vi "HFRR ADV v025 new software.vi"() -> ()   [LabVIEW 2025] (continued)
                    n3885 = local read item#-1() -> (w5335)
                    n3886 = Number To Fractional String(number=w5335, width (-)=i16 10, precision (6)=i16 4) -> (F-format string=w5339:string)  [unwired: 1 in]
                    n3887 = Concatenate Strings("LinearDeformation\":\"", w5339, w5337) -> (w5336:string)
                  }
                  frame #5 {
                    n3888 = local read "AIR TEMP"() -> (w5342:dbl)
                    n3889 = local read "Json St Flg"() -> (w5344:bool)
                    n3890 = local read "Json End Flg"() -> (w5345:bool)
                    n3891 = Number To Fractional String(number=w5342, width (-)=i16 10, precision (6)=i16 4) -> (F-format string=w5348:string)  [unwired: 1 in]
                    n3892 = Concatenate Strings("Vibration\":\"", w5348, w5346) -> (w5343:string)
                    n3893 = And(x=w5344, y=w5345) -> ()  [unwired: 1 out]
                  }
                  frame #6 {
                    n3894 = local read "Json End Flg"() -> (w5352:bool)
                    n3895 = Get Date/Time In Seconds() -> (seconds since 1Jan1904=w5360:timestamp)
                    n3896 = local read "Json St Flg"() -> (w5351:bool)
                    n3897 = To Double Precision Float(number=w5360) -> (double precision float=w5359:dbl)
                    n3898 = Subtract(x=w5359, y=2082844800.0) -> (x-y=w5357:dbl)
                    n3899 = Number To Fractional String(number=w5357, width (-)=i16 12, precision (6)=i16 0) -> (F-format string=w5354:string)  [unwired: 1 in]
                    n3900 = case shown="True" w5352 {
                      tunnel: ["" w5367] -> w5361
                      tunnel: w5354 -> [_ w5368]
                      tunnel: w5353 -> [_ w5366]
                      frame False {
                      }
                      frame True {
                        n3901 = local write "Json End Flg"(FALSE ("Json St Flg")) -> ()
                        n3902 = Concatenate Strings("End\": \"", w5368, w5366) -> (w5367:string)
                      }
                    }
                    n3903 = case shown="True" w5351 {
                      tunnel: [w5371 w5374] -> w5362
                      tunnel: w5354 -> [_ w5375]
                      tunnel: w5353 -> [_ w5372]
                      frame False {
                        n3904 = local read "St Str"() -> (w5371:string)
                      }
                      frame True {
                        n3905 = Concatenate Strings("Start\":\"", w5375, w5372) -> (w5374:string)
                        "St Str" <- w5374
                        n3906 = local write "Json St Flg"(FALSE ("Json St Flg")) -> ()
                      }
                    }
                    n3907 = Concatenate Strings(w5362, w5361, w5364) -> (w5363:string)
                  }
                }
                n3908 = local read "FILE"() -> (w5232:string)
                n3909 = Concatenate Strings("\",\"OperatorID\":\"" ("string"), "Operator ID") -> (w5235:string)
                n3910 = Concatenate Strings("\",\"DatasetTitle\":\"" ("string"), w5232) -> (w5234:string)
                n3911 = Concatenate Strings("\",\"SerialNumber\":\"" ("string"), "Serial No") -> (w5264:string)
                n3912 = Concatenate Strings("\",\"ModelNumber\":\"" ("string"), "Model No") -> (w5263:string)
                n3913 = Concatenate Strings(w5264, w5263) -> (w5246:string)
                n3914 = Concatenate Strings("{\"SecretKey\":\"", "Secret Key", w5246, w5235, w5234, "\",\"Samples\":[") -> (w5251:string)
                n3915 = Concatenate Strings(w5253, w5257, w5256, w5255, w5254, w5238, w5239, w5240) -> (w5252:string)
                n3916 = Concatenate Strings(w5251, w5252, "]}") -> (w5250:string)
                n3917 = stacked-sequence {
                  tunnel: w5250 -> [w5279 _ _]
                  tunnel: [_ _ w5296] -> _
                  frame #0 {
                    (unwired) FALSE ("convert eol (F)")
                    w5281 = enum16{"start", "end", "current"}."start" ("pos mode (0:2)")
                    n3918 = Path To String(path="Path") -> (string=w5287:string)
                    n3919 = Concatenate Strings(w5287, "\\", "Data File Name") -> (w5289:string)
                    n3920 = local write "standard output"(" ") -> ()
                    n3921 = String To Path(string=w5289) -> (path=w5278:path)
                    n3922 = call <vilib>:"Open_Create_Replace File.vi"("advisory dialog? (display:T)"=FALSE, "function (open:0)"=T30."create or replace", "file path"=w5278) -> ("error out"=w5292:errorcluster, "refnum"=w5291:refnum<file>)  [unwired: 5 in, 2 out]
                    n3923 = Set File Position(refnum=w5291, from (0:start)=w5281, error in=w5292) -> (refnum out=w5272:refnum<file>, error out=w5271:errorcluster)  [unwired: 1 in]
                    n3924 = Write to Binary File(file (use dialog)=w5272, data=" ", error in=w5271, 5:FALSE ("prepend array or string size? (T)")) -> (refnum out=w5282:refnum<file>, error out=w5283:errorcluster)  [unwired: 2 in, 1 out]
                    n3925 = Set File Position(offset (in bytes) (0)=w5281, refnum=w5282, error in=w5283) -> (refnum out=w5275:refnum<file>, error out=w5274:errorcluster)  [unwired: 1 in]
                    n3926 = Write to Binary File(file (use dialog)=w5275, data=w5279, error in=w5274, 5:FALSE ("prepend array or string size? (T)")) -> (error out=w5277:errorcluster)  [unwired: 2 in, 2 out]
                    n3927 = flat-sequence {
                      tunnel: w5278 -> [w5294]
                      tunnel: w5277 -> [_]
                      frame #0 {
                        n3928 = call <vilib>:"Read Characters From File.vi"("file path (dialog if empty)"=w5294) -> ("character string"=→"JSON string":string)  [unwired: 5 in, 3 out]
                      }
                    }
                    "SinglePoint" <- w5279
                  }
                  frame #1 {
                  }
                  frame #2 {
                    (unwired) "\"Stored\": true" ("string")
                    n3929 = call <vilib>:"System Exec.vi"("run minimized? (F)"=TRUE, "wait until completion? (T)"=TRUE, "working directory"=path "C:/LAB-IQ-NXT", "command line"="C:\\LAB-IQ-NXT\\JPost.bat") -> ("standard error"=→"Respose From Server":string, "standard output"=w5299:string)  [unwired: 4 in, 2 out]
                    "standard output" <- w5299
                    n3930 = Match Pattern(string=w5299, regular expression="JSON Check String") -> (match substring=w5297:string, offset past match=w5296:i32)  [unwired: 1 in, 2 out]
                    n3931 = Equal?(x=w5297, y="JSON Check String") -> (x = y?=→"Upload \nConfirmed":bool)
                  }
                }
              }
            }
            n3932 = local read "Quit"() -> (w5220:bool)
          }
        }
      }
    }
    frame Enabled {
    }
  }
  n3933 = disable-structure shown="Disabled" {
    disable-tunnel: _ -> [w5382 _]
    frame Disabled {
      n3934 = while {
        shift-right: [w5390] -> w5378
        shift-left: _ -> [w5391]
        shift-right: [w5388] -> w5379
        shift-left: errorcluster {"status"=TRUE, "code"=0, "source"="Init"} ("error out") -> [w5389]
        shift-right: [w5386] -> _
        shift-left: "" -> [w5387]
        tunnel: [w5384] -> _
        tunnel: w5382 -> [_]
        i -> [w5384]
        stop <- w5383 stop-if-true
        n3935 = flat-sequence {
          tunnel: [w5392] -> w5385
          frame #0 {
            n3936 = Wait (ms)(milliseconds to wait=10.0 ("Delay")) -> (millisecond timer value=w5392:u32)
          }
        }
        n3937 = case shown="No Error" w5389 {
          selector: w5389 -> [w5422 w5541]
          tunnel: [w5405 w5543] -> w5390
          tunnel: [w5404 w5542] -> w5388
          tunnel: w5391 -> [w5423 w5535]
          tunnel: w5387 -> [w5403 w5534]
          tunnel: [w5402 w5534] -> w5386
          tunnel: w5385 -> [_ _]
          frame No Error {
            n3938 = Concatenate Strings("\r", "\n") -> (w5414:string)  [unwired: 1 in]
            n3939 = case shown="True" w5415 {
              tunnel: w5423 -> [w5447 w5454]
              tunnel: w5422 -> [w5446 w5453]
              tunnel: [w5447 w5452] -> w5421
              tunnel: [w5446 w5451] -> w5401
              tunnel: w5414 -> [_ w5450]
              frame False {
              }
              frame True {
                n3940 = VISA Write(VISA resource name=w5454, write buffer=w5450, error in (no error)=w5453) -> (VISA resource name out=w5452:refnum<visa-resource-name>, error out=w5451:errorcluster)  [unwired: 1 out]
                n3941 = local write "Read String"("") -> ()
                n3942 = local write item#-1(FALSE) -> ()
              }
            }
            n3943 = property class="Instr"(reference=w5421, error in=w5401) -> (reference out=w5420:refnum<visa-resource-name>, error out=w5419:errorcluster, "Serial Settings:Number of Bytes at Serial Port"=w5418:u32)
            n3944 = Greater?(x=w5418, y=u32 100) -> (0:w5416:bool)
            n3945 = case shown="True" w5416 {
              tunnel: w5420 -> [w5457 w5481]
              tunnel: w5419 -> [w5456 w5480]
              tunnel: w5418 -> [_ w5479]
              tunnel: [w5457 w5478] -> w5407
              tunnel: [w5456 w5477] -> w5406
              tunnel: w5403 -> [w5455 w5476]
              tunnel: [w5455 ""] -> w5402
              frame False {
              }
              frame True {
                w5466 = u32 6 ("y")
                # "Page 84 of \nmanual"
                n3946 = VISA Read(VISA resource name=w5481, byte count=w5479, error in (no error)=w5480) -> (VISA resource name out=w5478:refnum<visa-resource-name>, read buffer=w5474:string, error out=w5477:errorcluster)  [unwired: 1 out]
                n3947 = while {
                  tunnel: w5474 -> [w5530]
                  tunnel: [w5526] -> w5468 mode=indexing
                  tunnel: [w5520] -> w5472 mode=indexing
                  tunnel: [w5518] -> _
                  i -> [w5518]
                  stop <- w5523 stop-if-true
                  n3948 = String Subset(string=w5530, offset (0)=w5518) -> (substring=w5525:string)  [unwired: 1 in]
                  n3949 = String To Byte Array(string=w5525) -> (unsigned byte array=w5529:u8[])
                  n3950 = String Length(string=w5525) -> (length=w5524:i32)
                  n3951 = Index Array(array=w5529) -> (element=w5528:u8)  [unwired: 1 in]
                  n3952 = Equal To 0?(x=w5524) -> (x = 0?=w5523:bool)
                  n3953 = Number To Boolean Array(number=w5528) -> (Boolean array=w5522:bool[])
                  n3954 = Reverse 1D Array(array=w5522) -> (reversed array=w5521:bool[])
                  n3955 = And(x=w5522, y=bool[] [FALSE, FALSE, FALSE, FALSE, FALSE, FALSE, TRUE, TRUE] ("Boolean array")) -> (x .and. y?=w5526:bool[])
                  n3956 = And(x=w5521, y=bool[] [FALSE, FALSE, TRUE, TRUE, TRUE, TRUE, TRUE, TRUE] ("Boolean array")) -> (x .and. y?=w5520:bool[])
                }
                n3957 = Concatenate Strings(w5476, w5474) -> (→"Read String":string)
                n3958 = while {
                  tunnel: w5468 -> [w5517] mode=indexing
                  tunnel: [w5513] -> w5471
                  i -> [w5513]
                  stop <- w5514 stop-if-true
                  n3959 = Search 1D Array(1D array=w5517, element=TRUE) -> (index of element=w5515:i32)  [unwired: 1 in]
                  n3960 = Less Than 0?(x=w5515) -> (x < 0?=w5514:bool)
                }
                n3961 = Delete From Array(array=w5472, length=w5471, index (row)=0) -> (array with subset deleted=w5467:bool[][])  [unwired: 1 in, 1 out]
                n3962 = Array Size(array=w5467) -> (size(s)=w5469:i32[])
                n3963 = Index Array(array=w5469) -> (element=w5461:i32)  [unwired: 1 in]
                n3964 = Greater?(x=w5461, y=w5466) -> (0:w5464:bool)
                n3965 = Subtract(x=w5461, y=w5466) -> (x-y=w5465:u32)
                n3966 = Select(t=w5465, s=w5464, f=u32 0) -> (s? t:f=w5462:u32)
                n3967 = while {
                  tunnel: w5467 -> [w5500]
                  tunnel: [w5502] -> w5460 mode=indexing
                  tunnel: w5462 -> [w5484]
                  i -> [w5501]
                  stop <- w5499 stop-if-true
                  w5491 = 6 ("index")
                  w5490 = 2 ("length")
                  # "Page 65 of \nmanual"
                  n3968 = Multiply(x=u32 3 ("y"), y=w5501) -> (x*y=w5498:u32)
                  n3969 = Divide(x=u32 102 ("y"), y=u32 65520) -> (x/y=w5508:dbl)
                  n3970 = Greater Or Equal?(x=w5498, y=w5484) -> (x >= y?=w5499:bool)
                  n3971 = Index Array(array=w5500, index (row) #1=w5498) -> (element #1=w5496:bool[], element #2=w5495:bool[], element #3=w5494:bool[])  [unwired: 5 in]
                  n3972 = Reverse 1D Array(array=w5496) -> (reversed array=w5489:bool[])
                  n3973 = Reverse 1D Array(array=w5495) -> (reversed array=w5493:bool[])
                  n3974 = Reverse 1D Array(array=w5494) -> (reversed array=w5492:bool[])
                  n3975 = Delete From Array(array=w5489, length=w5490, index=w5491) -> (array with subset deleted=w5485:bool[])  [unwired: 1 out]
                  n3976 = Delete From Array(array=w5493, length=w5490, index=w5491) -> (array with subset deleted=w5486:bool[])  [unwired: 1 out]
                  n3977 = Delete From Array(array=w5492, length=w5490, index=w5491) -> (array with subset deleted=w5487:bool[])  [unwired: 1 out]
                  n3978 = Insert Into Array(array=bool[] [] ("Boolean array"), new element #1=w5485, new element #2=w5486, new element #3=w5487) -> (w5488:bool[])  [unwired: 1 in]
                  n3979 = Boolean Array To Number(Boolean array=w5488) -> (number=w5497:u32)
                  n3980 = Multiply(x=w5508, y=w5497) -> (x*y=w5507:dbl)
                  n3981 = Decrement(x=w5507) -> (x-1=w5506:dbl)
                  n3982 = Divide(x=w5506, y=u32 100) -> (x/y=w5504:dbl)
                  n3983 = Multiply(x=w5504, y=u32 10) -> (x*y=w5502:dbl)
                }
                n3984 = Delete From Array(array=w5460) -> (array with subset deleted=w5459:dbl[])  [unwired: 2 in, 1 out]
                "Waveform Graph 5" <- w5459
                "Waveform Chart 3" <- w5459
                n3985 = call-poly <vilib>:"Mean.vi"("X"=w5459) -> ("mean"=w5458:dbl)  [unwired: 1 out]
                n3986 = case shown="True" {
                  selector: _ -> [_ _]
                  tunnel: w5458 -> [_ w5483]
                  frame False {
                  }
                  frame True {
                    n3987 = local write item#-1(FALSE ("Zero 4")) -> ()
                    "z_measure" <- w5483
                  }
                }
              }
            }
            n3988 = local read item#-1() -> (w5398)
            n3989 = local read item#-1() -> (w5397)
            n3990 = local read item#-1() -> (w5399)
            n3991 = local read item#-1() -> (w5396)
            n3992 = case shown="True" w5394 {
              tunnel: w5398 -> [_ w5426]
              tunnel: w5399 -> [_ w5425]
              frame False {
              }
              frame True {
                n3993 = Build Array(w5426, w5425) -> (w5424:void[])
                n3994 = local read item#-1() -> (w5429)
                n3995 = Build Array (concatenate)(w5429, w5424) -> (w5427:void[])
                n3996 = local write item#-1(w5427) -> ()
                n3997 = local write item#-1(FALSE ("Boolean 8")) -> ()
              }
            }
            n3998 = call "Build XY Graph"("Enable"=w5396, "Reset"=w5397, "Y Input"=w5399, "X Input"=w5398) -> ("XY Graph"=w5395:cluster{"Y":dbl[], "Y":dbl[]}[])  [unwired: 6 in, 1 out]
            n3999 = case shown="True" {
              selector: _ -> [_ _]
              frame False {
              }
              frame True {
                n4000 = local read item#-1() -> (w5430)
                n4001 = Index Array(array=w5430, index (col) #1=0 ("disabled index (col)"), index (col) #2=1 ("index (col)")) -> (element #1=w5432, element #2=w5431)  [unwired: 2 in]
                n4002 = call <vilib>:"Linear Fit.vi"("Y"=w5432, "X"=w5431) -> ()  [unwired: 9 in, 5 out]
                n4003 = local write item#-1(FALSE ("Boolean 9")) -> ()
              }
            }
            n4004 = case shown="True" {
              selector: _ -> [_ _]
              frame False {
              }
              frame True {
                n4005 = local write item#-1(dbl[][] [] ("Captured Values")) -> ()
                n4006 = local write item#-1(FALSE ("Boolean 7")) -> ()
              }
            }
            n4007 = Concatenate Strings("\r", "\n") -> (w5409:string, w5408:string)
            n4008 = case shown="True" w5400 {
              tunnel: w5407 -> [w5439 w5445]
              tunnel: w5406 -> [w5438 w5444]
              tunnel: [w5439 w5443] -> w5405
              tunnel: [w5438 w5442] -> w5404
              tunnel: w5409 -> [_ w5441]
              frame False {
              }
              frame True {
                n4009 = VISA Write(VISA resource name=w5445, write buffer=w5441, error in (no error)=w5444) -> (VISA resource name out=w5443:refnum<visa-resource-name>, error out=w5442:errorcluster)  [unwired: 1 out]
                n4010 = local write item#-1(FALSE ("WRITE")) -> ()
              }
            }
          }
          frame Error {
            w5533 = u16 10 items=["1.0"=10, "1.5"=15, "2.0"=20] ("stop bits (10: 1 bit)")
            n4011 = Wait (ms)(milliseconds to wait=u32 20) -> ()  [unwired: 1 out]
            n4012 = VISA Close(VISA resource name=w5535, error in (no error)=w5541) -> (error out=w5540:errorcluster)
            n4013 = call <vilib>:"Clear Errors.vi"("error in (no error)"=w5540) -> ("error out"=w5539:errorcluster)  [unwired: 5 in, 1 out]
            n4014 = call-poly "VISA Configure Serial Port"("timeout (10sec)"=u32 200, "Enable Termination\nChar (T)"=TRUE ("Enable Termination\nChar (T)"), "baud rate (9600)"=u32 921600, "error in (no error)"=w5539, "stop bits (10: 1 bit)"=w5533) -> ("VISA resource name"=w5531:refnum<visa-resource-name>, "VISA resource name out"=w5543:refnum<visa-resource-name>, "error out"=w5542:errorcluster)  [unwired: 8 in]
          }
        }
        n4015 = local read "Quit"() -> (w5383:bool)
      }
      n4016 = VISA Close(VISA resource name=w5378, error in (no error)=w5379) -> (error out=w5377:errorcluster)
      n4017 = call <vilib>:"Clear Errors.vi"("error in (no error)"=w5377) -> ()  [unwired: 5 in, 2 out]
    }
    frame Enabled {
    }
  }
  n4018 = disable-structure shown="Disabled" {
    disable-tunnel: _ -> [w5548 _]
    frame Disabled {
      n4019 = while {
        tunnel: [w5555] -> _
        shift-right: [w5552] -> w5545
        shift-left: _ -> [w5554]
        shift-right: [w5553] -> w5546
        shift-left: errorcluster {"status"=TRUE, "code"=0, "source"="Init"} ("error out") -> [w5551]
        tunnel: w5548 -> [_]
        i -> [w5555]
        stop <- w5549 stop-if-true
        n4020 = flat-sequence {
          tunnel: w5551 -> [w5646]
          tunnel: [w5646] -> w5550
          frame #0 {
            n4021 = Wait (ms)(milliseconds to wait=u32 50) -> ()  [unwired: 1 out]
          }
        }
        n4022 = case shown="No Error" w5550 {
          selector: w5550 -> [w5596 w5639]
          tunnel: w5554 -> [w5595 w5638]
          tunnel: [w5562 w5629] -> w5553
          tunnel: [w5563 w5637] -> w5552
          frame No Error {
            w5589 = T31 {"Mode"=enum."RTU", "Slave Address"=1} ("Serial Parameters")
            n4023 = call-poly <vilib>:"MB Serial Master Query (poly).vi"("VISA resource name"=w5595, "Starting Address"=i16 1000, "Quantity"=u16 1, "Timeout"=u32 1000, "error in"=w5596, "Serial Parameters"=w5589) -> ("VISA resource name out"=w5590:refnum<visa-resource-name>, "Input Registers"=w5592:u16[], "error out"=w5588:errorcluster)  [unwired: 10 in, 1 out]
            n4024 = Random Number (0-1)() -> (number: 0 to 1=w5577:dbl)
            n4025 = Index Array(array=w5592, index=0) -> (element=w5587:u16)
            n4026 = Subtract(x=w5577, y=0.5) -> (x-y=w5576:dbl)
            n4027 = Divide(x=w5587, y=10 ("index")) -> (x/y=w5581:dbl)
            n4028 = Multiply(x=w5576, y=0.5) -> (x*y=w5575:dbl)
            n4029 = Add(x=w5581, y=w5575) -> (x+y=w5580:dbl)
            n4030 = local read "Amb temp"() -> (w5564:dbl)
            n4031 = Multiply(x=w5580, y=0.2) -> (x*y=w5584:dbl)
            n4032 = Multiply(x=w5564, y=0.8) -> (x*y=w5582:dbl)
            n4033 = Add(x=w5584, y=w5582) -> (x+y=w5565:dbl)
            n4034 = local read "set temp old"() -> (w5559:dbl)
            n4035 = local write "Amb temp"(w5565) -> ()
            n4036 = Select(t="SetTemp 2", s="Heater", f=100.0) -> (s? t:f=w5560:dbl)
            n4037 = Not Equal?(x=w5560, y=w5559) -> (x != y?=w5558:bool)
            n4038 = case shown="True" w5558 {
              tunnel: w5590 -> [w5624 w5626]
              tunnel: [w5623 w5626] -> w5570
              tunnel: w5588 -> [w5622 w5625]
              tunnel: [w5621 w5625] -> w5568
              tunnel: w5560 -> [w5616 _]
              tunnel: w5589 -> [w5618 w5627]
              tunnel: [w5618 w5627] -> w5571
              frame True {
                n4039 = Multiply(x=w5616, y=10 ("index")) -> (x*y=w5615:dbl)
                n4040 = call-poly <vilib>:"MB Serial Master Query (poly).vi"("VISA resource name"=w5624, "Address"=u16 0, "Holding Register"=w5615, "Timeout"=u32 1000, "error in"=w5622, "Serial Parameters"=w5618) -> ("VISA resource name out"=w5623:refnum<visa-resource-name>, "error out"=w5621:errorcluster)  [unwired: 11 in, 1 out]
                "set temp old" <- w5616
              }
              frame False {
              }
            }
            n4041 = flat-sequence {
              tunnel: [w5597] -> _
              tunnel: [w5597] -> w5567
              tunnel: w5568 -> [w5597]
              frame #0 {
                n4042 = Wait (ms)(milliseconds to wait=u32 100) -> ()  [unwired: 1 out]
              }
            }
            n4043 = call "Elapsed Time12"("Time Target (s)"=2.0, "Auto Reset"=TRUE) -> ("Time has Elapsed"=w5572:bool)  [unwired: 10 in, 7 out]
            n4044 = case shown="True" w5572 {
              tunnel: w5571 -> [w5601 w5614]
              tunnel: [w5601 w5614] -> _
              tunnel: [w5600 w5612] -> w5563
              tunnel: w5570 -> [w5600 w5613]
              tunnel: [w5599 w5610] -> w5562
              tunnel: w5567 -> [w5599 w5611]
              frame False {
              }
              frame True {
                n4045 = call-poly <vilib>:"MB Serial Master Query (poly).vi"("VISA resource name"=w5613, "Starting Address"=i16 1003 ("Addr"), "Quantity"=u16 1, "Timeout"=u32 1000, "error in"=w5611, "Serial Parameters"=w5614) -> ("VISA resource name out"=w5612:refnum<visa-resource-name>, "Input Registers"=w5607:u16[], "error out"=w5610:errorcluster)  [unwired: 10 in, 1 out]
                n4046 = Index Array(array=w5607, index=0) -> (element=w5606:u16)
                n4047 = Divide(x=w5606, y=u16 10) -> (x/y=w5602:dbl)
                n4048 = local write "set temp old"(w5602) -> ()
                n4049 = local write "SetTemp"(w5602) -> ()
              }
            }
            "Error Code" <- w5562
            n4050 = Unbundle(w5562) -> ("status"=→"TK4 status":bool)  [unwired: 2 out]
            "SetTemp" <- "SetTemp 2"
          }
          frame Error {
            w5641 = u16 0 items=["None", "Odd", "Even", "Mark", "Space"] ("Parity")
            w5642 = u16 0 items=["None", "XON/XOFF", "RTS/CTS", "XON/XOFF & RTS/CTS", "DTR/DSR", "XON/XOFF & DTR/DSR"] ("Flow Control")
            n4051 = VISA Clear(VISA resource name=w5638, error in (no error)=w5639) -> (VISA resource name out=w5632:refnum<visa-resource-name>, error out=w5630:errorcluster)
            n4052 = VISA Close(VISA resource name=w5632, error in (no error)=w5630) -> (error out=w5631:errorcluster)
            n4053 = call <vilib>:"Clear Errors.vi"("error in (no error)"=w5631) -> ("error out"=w5640:errorcluster)  [unwired: 5 in, 1 out]
            n4054 = Unbundle By Name(T31 {"Mode"=enum."RTU", "Slave Address"=1} ("input cluster")) -> ("Mode"=w5643:enum16{"RTU", "ASCII"})
            n4055 = call <vilib>:"MB Serial Init.vi"("Timeout"=u32 100, "Flow Control"=w5642, "Mode"=w5643, "error in (no error)"=w5640, "Parity"=w5641, "Baud Rate"=u32 9600, "VISA resource name"="Lubrication System COM Port :") -> ("error out"=w5629:errorcluster, "VISA resource name out"=w5637:refnum<visa-resource-name>)  [unwired: 3 in]
            n4056 = local write "set temp old"(0.0 ("set temp old")) -> ()
            n4057 = Unbundle(w5629) -> ("status"=w5628:bool)  [unwired: 2 out]
            n4058 = case shown="True" w5628 {
              selector: w5628 -> [_ w5645]
              frame False {
              }
              frame True {
                n4059 = local write "TK4 status"(w5645) -> ()
              }
            }
          }
        }
        n4060 = local read "Quit"() -> (w5549:bool)
      }
      n4061 = VISA Close(VISA resource name=w5545, error in (no error)=w5546) -> (error out=w5544:errorcluster)
      n4062 = call <vilib>:"Clear Errors.vi"("error in (no error)"=w5544) -> ()  [unwired: 5 in, 2 out]
    }
    frame Enabled {
    }
  }
